vi "SVMabcSGL_src.vi"(0 "A":sgl, 1 "max":sgl=0.9999695 caption="max voltage", 5 "B":sgl, 7 "C":sgl) -> (4 "Upercent":sgl caption="u voltage" format="%.21g", 6 "Vpercent":sgl caption="v voltage" format="%.21g", 8 "Wpercent":sgl caption="w voltage" format="%.21g", 15 "Sector":u8)   [LabVIEW 2015]
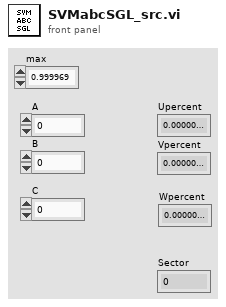
[diagram p1: front panel]
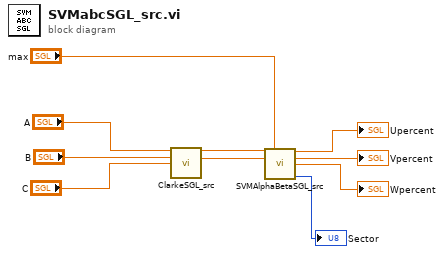
[diagram p0: block diagram]
diagram:
  n1 = call "ClarkeSGL_src.vi"("A"="A", "B"="B", "C"="C") -> ("alpha"=w10:sgl, "beta"=w9:sgl)  [unwired: 11 in]
  n2 = call "SVMAlphaBetaSGL_src.vi"("alpha"=w10, "max"="max", "beta"=w9) -> ("Upercent"=→"Upercent":sgl, "Vpercent"=→"Vpercent":sgl, "Wpercent"=→"Wpercent":sgl, "Sector"=→"Sector":u8)  [unwired: 9 in]
